vi "_Parse Detected Modulation Segment.vi"(8 "error in (no error)":errorcluster, 10 "Input String":string, 11 "VISA resource name":refnum<visa-resource-name>) -> (0 "error out":errorcluster, 1 "Detected Modulation":i32, 2 "Reliability Results":T1, 3 "VISA resource name out":refnum<visa-resource-name>)   [LabVIEW 2020, in "Rohde&Schwarz CMXP NR FR2 Measurement.lvlib"]
uses:
  <instrlib>/Rohde&Schwarz CMXP NR FR2 Measurement/Rohde&Schwarz CMXP NR FR2 Measurement.lvlib
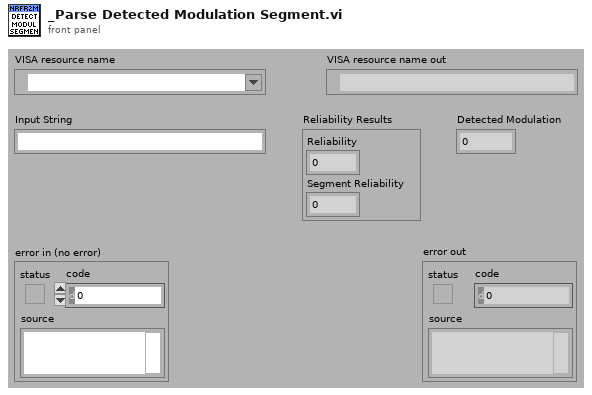
[diagram p1: front panel]
types:
  T1 = cluster{"Reliability":i32, "Segment Reliability":i32}
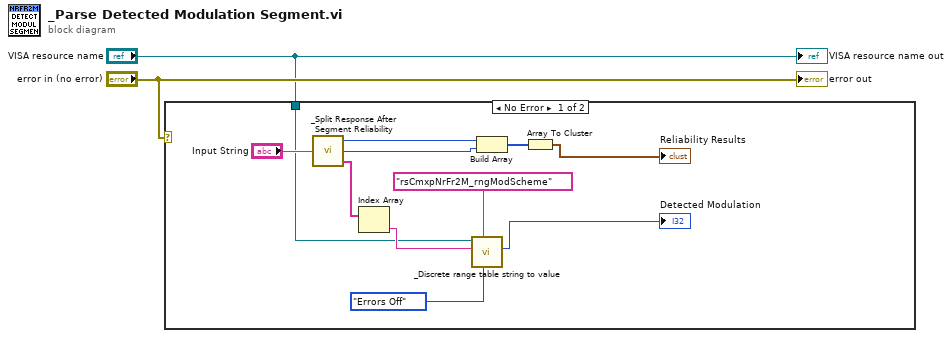
[diagram p0: block diagram]
diagram:
  n1 = case shown="No Error" "error in (no error)" {
    tunnel: "VISA resource name" -> [w3 _]
    frame No Error {
      n2 = call <instrlib>:"_Split Response After Segment Reliability.vi"("Input String"="Input String") -> ("Response out"=w6:string[], "Segment Reliability"=w10:i32, "Reliability"=w11:i32)
      n3 = Index Array(array=w6) -> (element=w5:string)  [unwired: 1 in]
      n4 = call <instrlib>:"_Discrete range table string to value.vi"("Error Mode (Warnings)"=enum16{"Errors Off", "Errors", "Warnings"}."Errors Off", "Discrete Range Table Identifier"="rsCmxpNrFr2M_rngModScheme", "String Value In"=w5, "VISA resource name"=w3) -> ("Enum Value"=→"Detected Modulation":i32)  [unwired: 5 in, 2 out]
      n5 = Build Array(w11, w10) -> (w9:i32[])
      n6 = Array To Cluster(array=w9) -> (cluster=→"Reliability Results":cluster{"[0]":i32, "[1]":i32})
    }
    frame Error {
    }
  }
  "VISA resource name out" <- "VISA resource name"
  "error out" <- "error in (no error)"
